vi "Analog Read.vi"   [LabVIEW 2014, in "LMH-LINX.lvlib"]
doc: "Read the value of the specified analog input channel(s)."
uses:
  <vilib>/MakerHub/LINX/LMH-LINX.lvlib
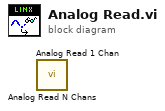
[diagram p0: block diagram]
diagram:
  n1 = call <vilib>:"Analog Read N Chans.vi"() -> ()  [unwired: 8 in, 4 out]
  n2 = call <vilib>:"Analog Read 1 Chan.vi"() -> ()  [unwired: 8 in, 4 out]
